vi "set_dc_supply (SubVI).vi"(11 "Tot DC Arr":dbl[](array[numeric])) -> (2 "Set DC?":bool, 3 "Agilent is \nplugged in \nnegative?":bool)   [LabVIEW 2016]
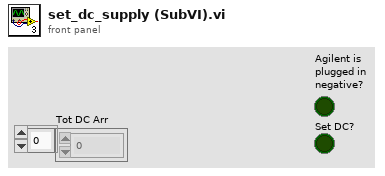
[diagram p1: front panel]
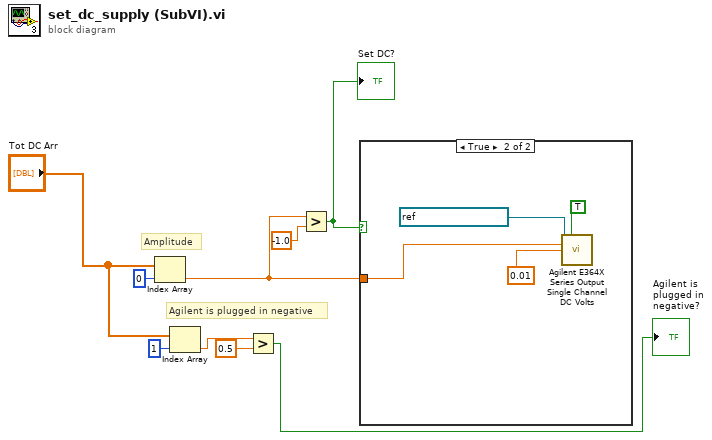
[diagram p0: block diagram]
diagram:
  # "Agilent is plugged in negative"
  # "Amplitude"
  n1 = Index Array(array="Tot DC Arr", index=0) -> (element=w3:dbl)
  n2 = Index Array(array="Tot DC Arr", index=1) -> (element=w6:dbl)
  n3 = Greater?(x=w6, y=0.5) -> (0:→"Agilent is \nplugged in \nnegative?":bool)
  n4 = Greater?(x=w3, y=-1.0) -> (0:w1:bool)
  "Set DC?" <- w1
  n5 = case shown="True" w1 {
    tunnel: w3 -> [_ w13]
    frame False {
    }
    frame True {
      n6 = call <instrlib>:"Agilent E364X Series Output Single Channel DC Volts.vi"("VISA resource name"=refnum<visa-resource-name> "GPIB0::8::INSTR", "Output Enabled (False)"=TRUE, "Voltage Level (0.0 Volts)"=w13, "Current Limit (0 Amps)"=0.01) -> ()  [unwired: 11 in, 1 out]
    }
  }
